vi "lfsr.vi"(1 "Input":u16) -> (0 "Output":u16)   [LabVIEW 2013]
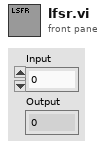
[diagram p1: front panel]
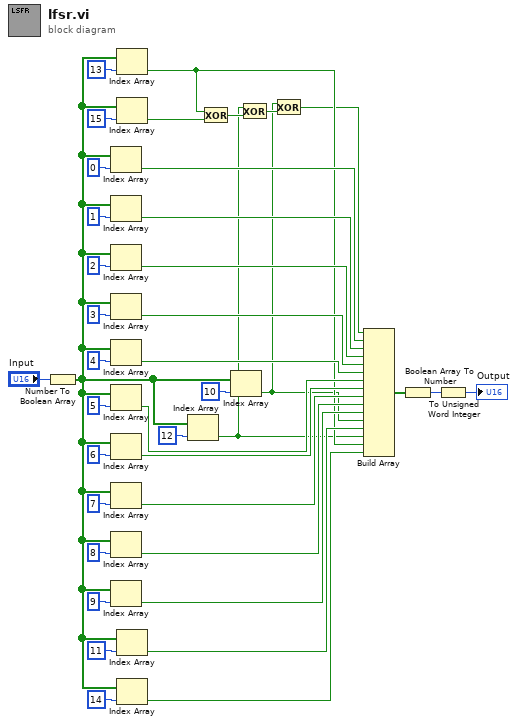
[diagram p0: block diagram]
diagram:
  n1 = Number To Boolean Array(number="Input") -> (Boolean array=w27:bool[])
  n2 = Index Array(array=w27, index=0) -> (element=w39:bool)
  n3 = Index Array(array=w27, index=1) -> (element=w38:bool)
  n4 = Index Array(array=w27, index=2) -> (element=w37:bool)
  n5 = Index Array(array=w27, index=3) -> (element=w36:bool)
  n6 = Index Array(array=w27, index=4) -> (element=w35:bool)
  n7 = Index Array(array=w27, index=5) -> (element=w34:bool)
  n8 = Index Array(array=w27, index=6) -> (element=w33:bool)
  n9 = Index Array(array=w27, index=7) -> (element=w32:bool)
  n10 = Index Array(array=w27, index=8) -> (element=w31:bool)
  n11 = Index Array(array=w27, index=9) -> (element=w30:bool)
  n12 = Index Array(array=w27, index=13) -> (element=w24:bool)
  n13 = Index Array(array=w27, index=15) -> (element=w23:bool)
  n14 = Index Array(array=w27, index=11) -> (element=w29:bool)
  n15 = Index Array(array=w27, index=14) -> (element=w28:bool)
  n16 = Index Array(array=w27, index=12) -> (element=w21:bool)
  n17 = Exclusive Or(1:w23, 2:w24) -> (0:w22:bool)
  n18 = Index Array(array=w27, index=10) -> (element=w19:bool)
  n19 = Exclusive Or(1:w22, 2:w21) -> (0:w20:bool)
  n20 = Exclusive Or(1:w20, 2:w19) -> (0:w18:bool)
  n21 = Build Array(w18, w39, w38, w37, w36, w35, w34, w33, w32, w31, w30, w19, w29, w21, w24, w28) -> (w26:bool[])
  n22 = Boolean Array To Number(Boolean array=w26) -> (number=w25:u32)
  n23 = To Unsigned Word Integer(number=w25) -> (unsigned 16bit integer=→"Output":u16)
